vi "Analyse Content.vi"(8 "error in (no error)":errorcluster, 11 "Content in":refnum<class "Content.lvclass">) -> (0 "error out":errorcluster, 3 "Content out":refnum<class "Content.lvclass">)   [LabVIEW 2026, in "LED Matrix.lvlib" / "Content.lvclass"]
uses:
  Content.lvclass
  Content.lvclass/Content.ctl
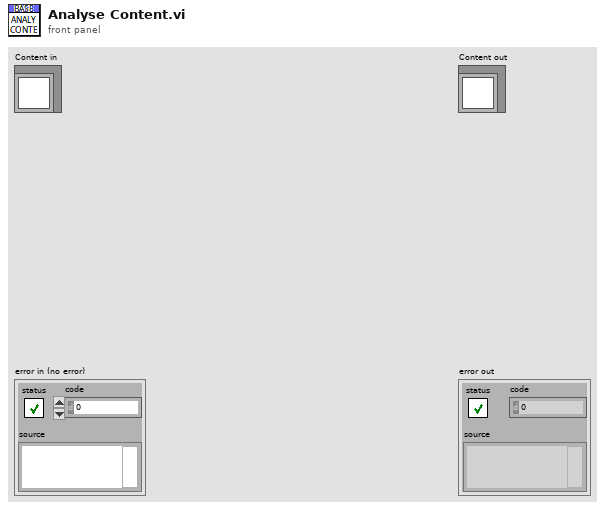
[diagram p1: front panel]
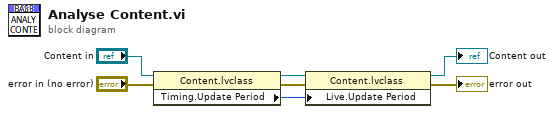
[diagram p0: block diagram]
diagram:
  n1 = property class="Content.lvclass"(reference="Content in", error in="error in (no error)") -> (reference out=w3:refnum<class "Content.lvclass">, error out=w6:errorcluster, "Timing.Update Period"=w1:i32)
  n2 = property class="Content.lvclass"(reference=w3, error in=w6, "Live.Update Period"=w1) -> (reference out=→"Content out":refnum<class "Content.lvclass">, error out=→"error out":errorcluster)
